vi "Test-Alert-Handler.vi"   [LabVIEW 2014]
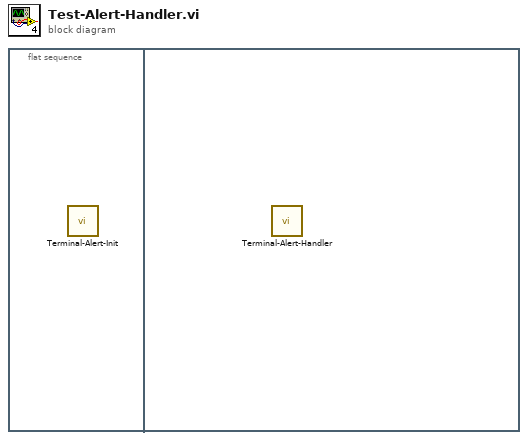
[diagram p0: block diagram]
diagram:
  n1 = flat-sequence {
    frame #0 {
      n2 = call "Terminal-Alert-Init.vi"() -> ()  [unwired: 12 in]
    }
    frame #1 {
      n3 = call "Terminal-Alert-Handler.vi"() -> ()  [unwired: 12 in]
    }
  }
